vi "createCommand.vi"(8 "error in (no error)":errorcluster, 9 "Variant":variant, 10 "commands":T1, 11 "AlCS in":refnum<class "AlCS.lvclass">) -> (0 "error out":errorcluster, 2 "command":string, 3 "AlCS out":refnum<class "AlCS.lvclass">)   [LabVIEW 2016, in "AlCS.lvclass"]
uses:
  AlCS.lvclass
  Typedefs/Commands.ctl
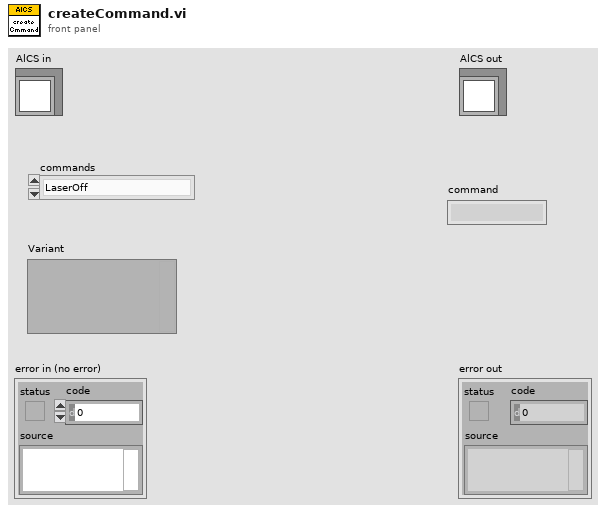
[diagram p1: front panel]
types:
  T1 = typedef "Commands.ctl" = enum16{"LaserOff", "MP", "queryStatus", "queryLaserStatus", "queryPosition", "clearError"}
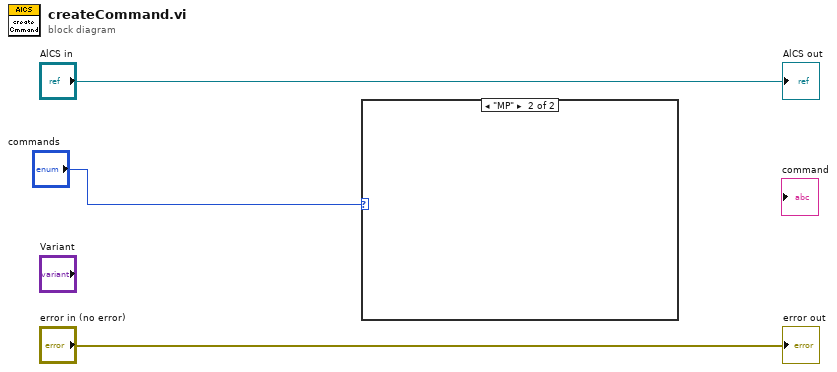
[diagram p0: block diagram]
diagram:
  n1 = case shown="\"MP\"" "commands" {
    frame "LaserOff", Default {
    }
    frame "MP" {
    }
  }
  "error out" <- "error in (no error)"
  "AlCS out" <- "AlCS in"
